vi "SQL Create Table.vi"(8 "error in":errorcluster, 10 "Primary Key?":bool, 11 "variant":variant) -> (0 "error out":errorcluster, 1 "Array":T2(array[cluster]), 3 "SQL QUERY":string)   [LabVIEW 2021]
uses:
  <vilib>/Utility/Data Type/Type Definitions/Data Type.ctl
  <vilib>/Utility/Data Type/NI_Data Type.lvlib
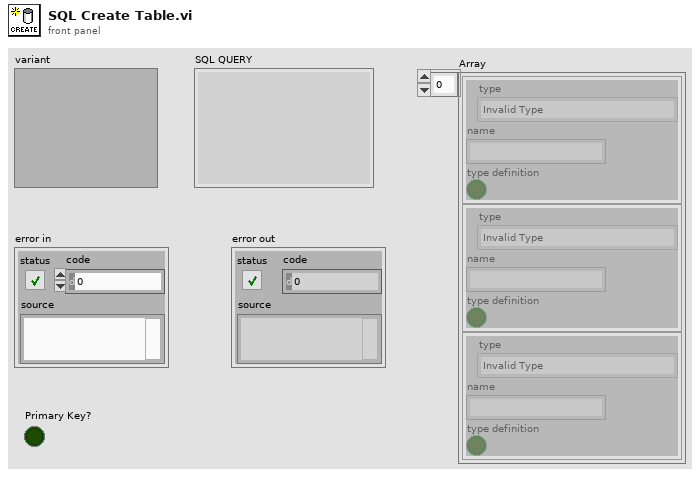
[diagram p1: front panel]
types:
  T1 = typedef "NI_Data Type.lvlib/Data Type.ctl" = enum8{"Invalid Type", "Void", "I8", "I16", "I32", "I64", "U8", "U16", "U32", "U64", "Single Float", "Double Float", "Extended Float", "Single Complex", "Double Complex", "Extended Complex", "Enum U8", "Enum U16", "Enum U32", "Enum U64", "Single Float With Unit", "Double Float With Unit", "Extended Float With Unit", "Single Complex with Unit", "Double Complex with Unit", "Extended Complex with Unit", "Boolean", "String", "Path", "Picture", "Tag", "Array", "Cluster", "Variant", "LV Variant", "Waveform", "Timestamp", "Digital Waveform", "Digital Data", "ExpressData", "Refnum", "External Data", "VI", "Poly VI", "LabVIEW Class Instance", "Fixed Point", "Set Collection", "Map Collection"}
  T2 = cluster{"type":T1, "name":string, "type definition":bool}[]
  T3 = cluster{"type":T1, "name":string, "type definition":bool}
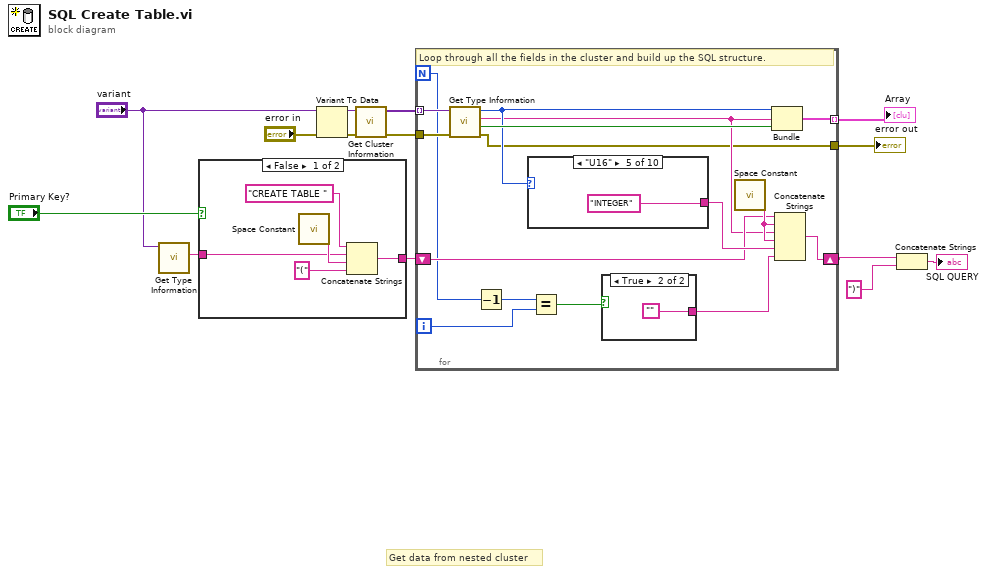
[diagram p0: block diagram]
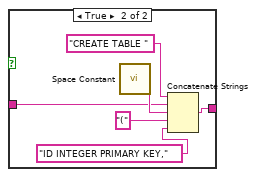
[diagram p2: hidden frame]
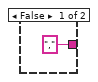
[diagram p3: hidden frame]
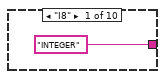
[diagram p4: hidden frame]
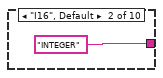
[diagram p5: hidden frame]
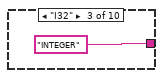
[diagram p6: hidden frame]
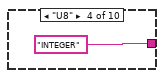
[diagram p7: hidden frame]
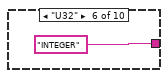
[diagram p8: hidden frame]
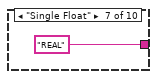
[diagram p9: hidden frame]
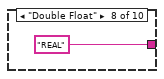
[diagram p10: hidden frame]
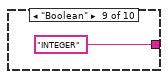
[diagram p11: hidden frame]
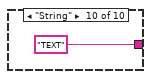
[diagram p12: hidden frame]
diagram:
  # "Get data from nested cluster"
  n1 = call <vilib>:"Get Type Information.vi"("variant"="variant") -> ("name"=w7:string)  [unwired: 6 in, 4 out]
  n2 = case shown="False" "Primary Key?" {
    tunnel: w7 -> [w16 w22]
    tunnel: [w15 w21] -> w6
    frame False {
      n3 = call <vilib>:"Space Constant.vi"() -> ("String"=w18:string)
      n4 = Concatenate Strings("CREATE TABLE " ("Table Name"), w16, w18, "(" ("Table Name")) -> (w15:string)
    }
    frame True {
      n5 = call <vilib>:"Space Constant.vi"() -> ("String"=w24:string)
      n6 = Concatenate Strings("CREATE TABLE " ("Table Name"), w22, w24, "(" ("Table Name"), "ID INTEGER PRIMARY KEY," ("string")) -> (w21:string)
    }
  }
  n7 = Variant To Data(error in="error in", Variant="variant") -> (data=w13:variant, error out=w14:errorcluster)  [unwired: 1 in]
  n8 = call <vilib>:"Get Cluster Information.vi"("error in (no error)"=w14, "variant"=w13) -> ("error out"=w12:errorcluster, "cluster elements"=w11:variant[])  [unwired: 8 in]
  n9 = for {
    N -> [w30]
    tunnel: w11 -> [w38] mode=indexing
    tunnel: w12 -> [w41]
    tunnel: [w39] -> w8 mode=indexing
    shift-right: [w36] -> w4
    shift-left: w6 -> [w33]
    tunnel: [w26] -> w9
    i -> [w32]
    # "Loop through all the fields in the cluster and build up the SQL structure."
    n10 = call <vilib>:"Get Type Information.vi"("error in (no error)"=w41, "variant"=w38) -> ("error out"=w26:errorcluster, "type definition"=w40:bool, "name"=w28:string, "type"=w37:T1)  [unwired: 5 in, 1 out]
    n11 = Decrement(x=w30) -> (x-1=w29:i32)
    n12 = case shown="\"U16\"" w37 {
      tunnel: ["INTEGER" "INTEGER" "INTEGER" "INTEGER" "INTEGER" "INTEGER" "REAL" "REAL" "INTEGER" "TEXT"] -> w35
      frame "I8" {
      }
      frame "I16", Default {
      }
      frame "I32" {
      }
      frame "U8" {
      }
      frame "U16" {
      }
      frame "U32" {
      }
      frame "Single Float" {
      }
      frame "Double Float" {
      }
      frame "Boolean" {
      }
      frame "String" {
      }
    }
    n13 = Equal?(x=w29, y=w32) -> (x = y?=w31:bool)
    n14 = case shown="True" w31 {
      tunnel: ["," ("delimiter (Tab)") ""] -> w27
      frame False {
      }
      frame True {
      }
    }
    n15 = call <vilib>:"Space Constant.vi"() -> ("String"=w34:string)
    n16 = Bundle("type"=w37, "name"=w28, "type definition"=w40) -> (w39:T3)  [unwired: 1 in]
    n17 = Concatenate Strings(w33, w34, w28, w34, w35, w27) -> (w36:string)
  }
  "error out" <- w9
  "Array" <- w8
  n18 = Concatenate Strings(w4, ")") -> (→"SQL QUERY":string)
